vi "SSS_V4_0.vi"() -> ()   [LabVIEW 2017]
uses:
  <vilib>/DAQmx/write.llb/DAQmx Write (Analog 2D DBL NChan NSamp).vi
  <vilib>/DAQmx/read.llb/DAQmx Read (Analog 1D Wfm NChan NSamp).vi
  <vilib>/DAQmx/create/channels.llb/DAQmx Create Channel (AO-Voltage-Basic).vi
  <vilib>/DAQmx/create/channels.llb/DAQmx Create Channel (AI-Voltage-Basic).vi
  <vilib>/DAQmx/configure/timing.llb/DAQmx Timing (Sample Clock).vi
  <vilib>/DAQmx/miscellaneous.llb/DAQmx Fill In Error Info.vi
  <vilib>/Analysis/3filter.llb/FIR Filter (DBL).vi
  <vilib>/Analysis/NI_AALBase.lvlib
panel:
  out "크기 3":i32
  out "부호없는 바이트 배열":u8[](array[numeric])
  in  "Server Closed 2":string="The server VI closed the connection."
  out "연결 ID":refnum<k5>
  out "Signal Processing Result 2":waveform(dbl)(graph)
  out "Signal Processing Result":waveform(dbl)(graph)
  out "크기":i32
  in  "physical channels":tag="Dev3/ao0:1" caption="송신 채널 설정"
  in  "Samplig Rate(RX)":dbl=1500000.0
  in  "RX time(sec)":dbl=0.1
  out "RX.CH2":waveform(dbl)(graph)
  out "RX.CH1":waveform(dbl)(graph)
  in  "Start Frequency(Hz)":dbl=430000.0 format="%#_6p"
  in  "Pulse length(sec)":dbl=0.0004
  in  "sampling rate(TX)":dbl=3760000.0 caption="Sampling Rate(TX)" format="%#.2g"
  in  "STEP":i32=100
  in  "초기 위상":dbl format="%#_13g"
  in  "Bandwidth":dbl=40000.0 format="%#_6p"
  out "Hz/1STEP":dbl
  out "TX.CH1":waveform(dbl)(graph)
  out "TX.CH 2":waveform(dbl)(graph)
  in  "수신 디바이스 이름":tag="Dev3"
  in  "수신 채널 설정":tag="Dev3/ai0:1"
  in  "송신 디바이스 이름":tag="Dev3"
  out "불리언 2":bool
  in  "Signal_Processing 2":bool
  out "CMD_PWD_DATA":i32=4
  in  "Signal_Processing":bool
  out "CMD_PWD":i32=7
  out "CMD_TVG":i32=6
  out "CMD_TVG_DATA":i32=4
  out "CMD_GAIN":i32=5
  out "CMD_GAIN_DATA":i32=255
  out "CMD_RANGE":i32=4
  out "CMD_RANGE_DATA":i32=100
  out "CMD_STOP":i32=3
  out "CMD_STOP_DATA":i32
  out "CMD_START":i32=2
  out "CMD_START_DATA":i32=1
  in  "port":u16=2500
  in  "address":string="30.0.1.18"
  in  "TCP/IP":bool
  in  "Server Closed":string="The server VI closed the connection."
  # "송신 신호 변조 설정"
  # "DAQ Max 설정"
  # "TCP/IP 소켓 통신 설정"
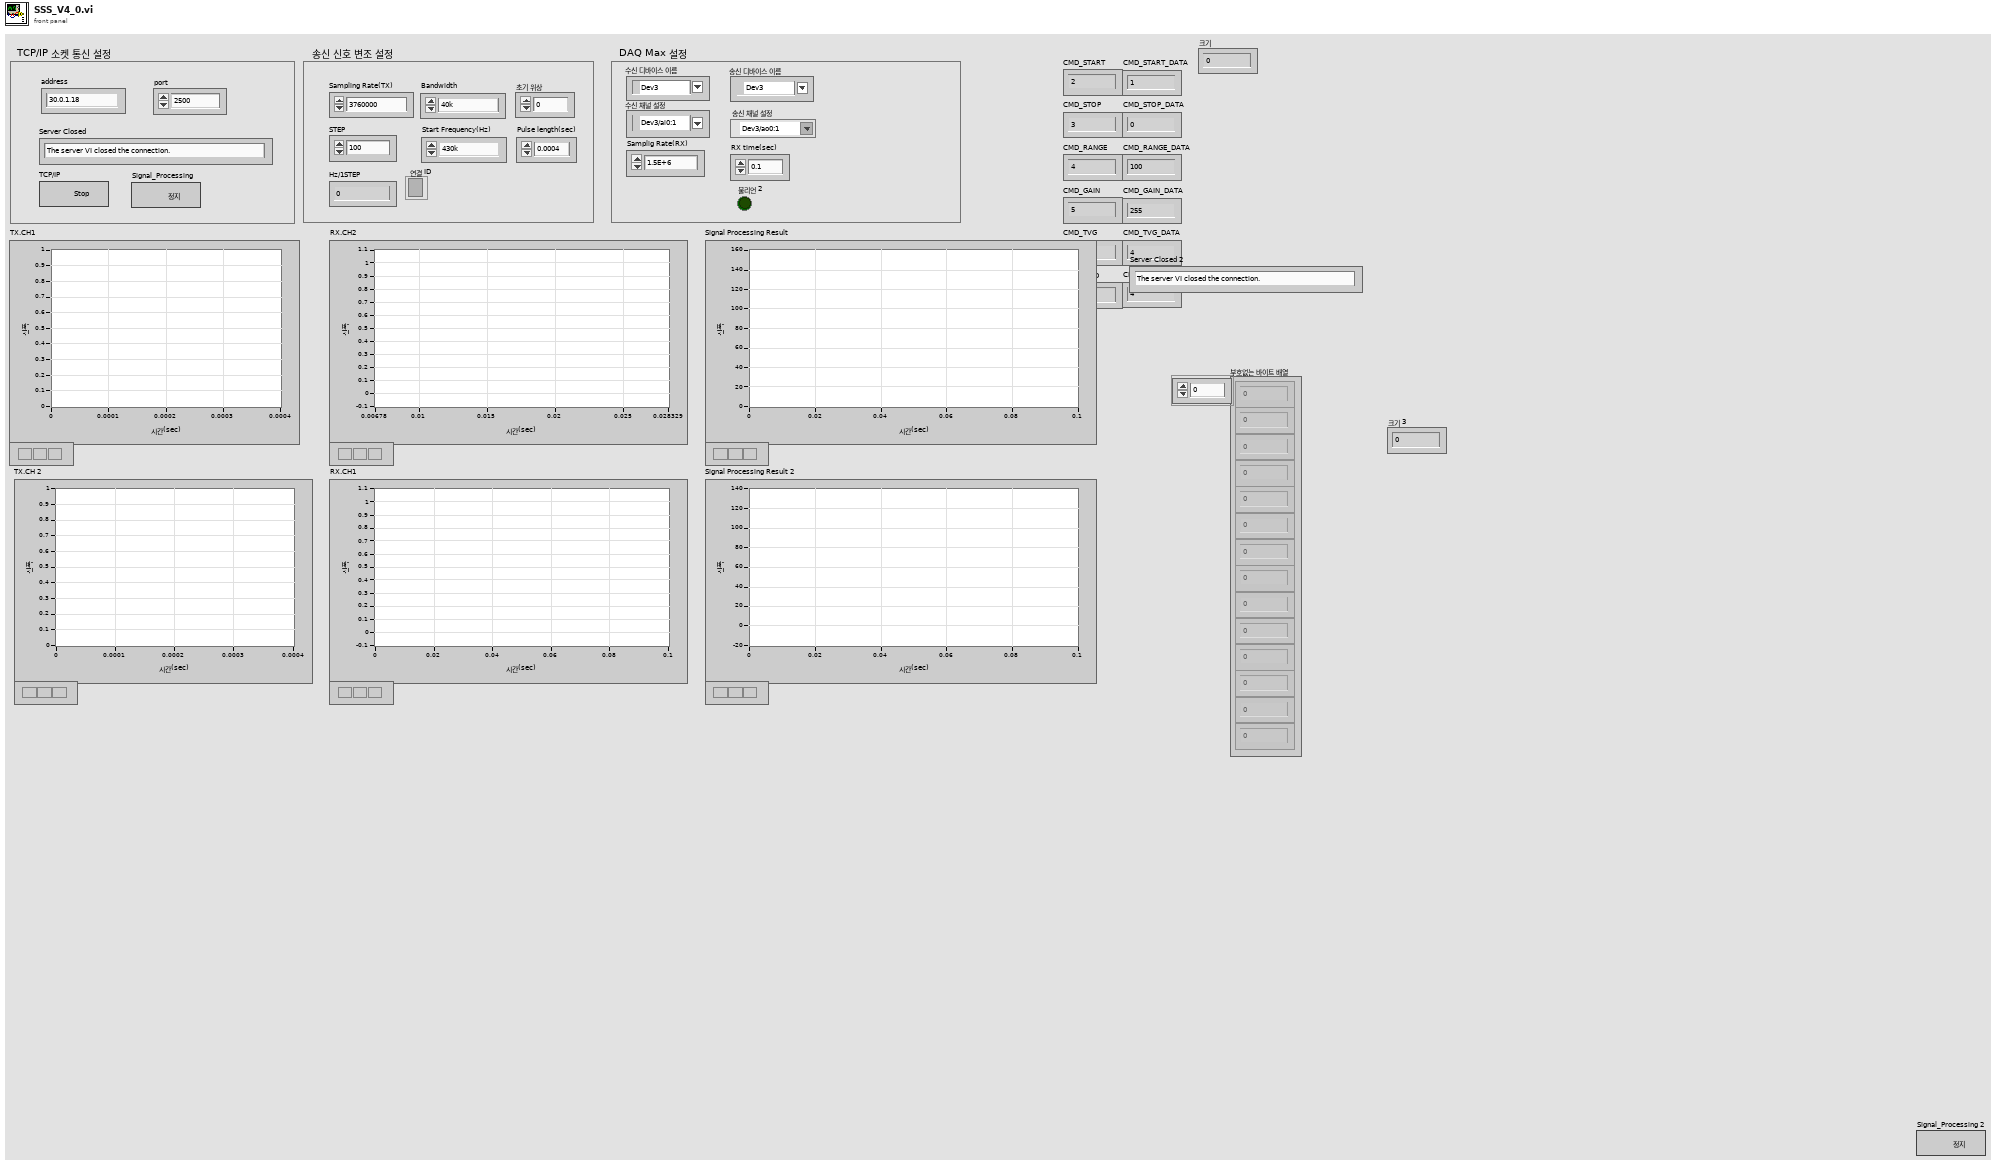
[diagram p1: front panel]
types:
  T1 = enum16{"Standard", "Buffered", "CRLF", "Immediate"}
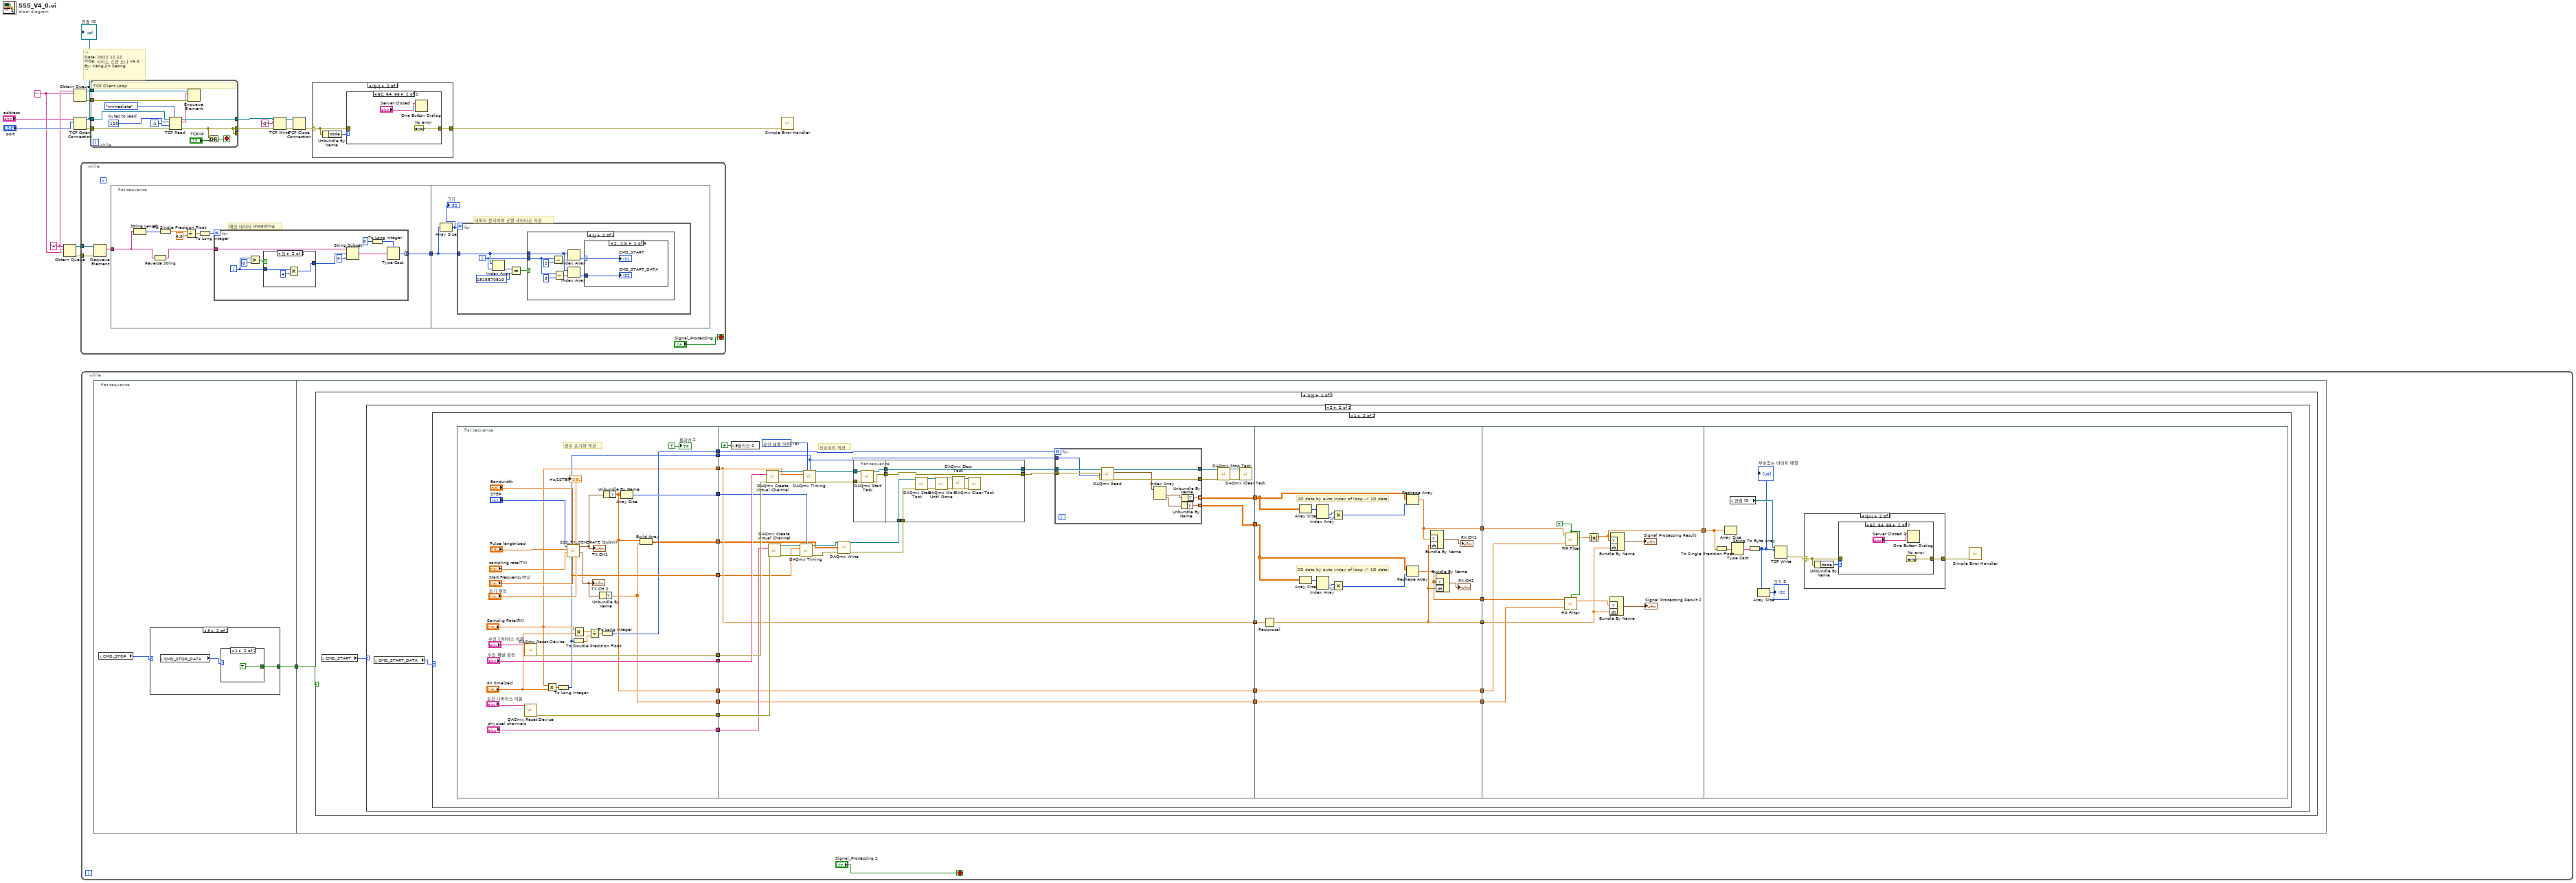
[diagram p0: block diagram]
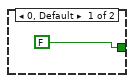
[diagram p2: hidden frame]
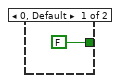
[diagram p3: hidden frame]
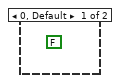
[diagram p4: hidden frame]
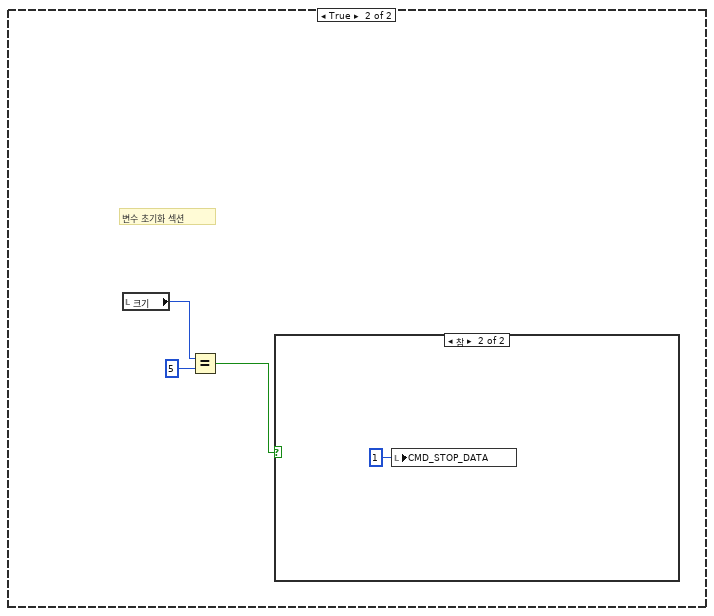
[diagram p8: hidden frame]
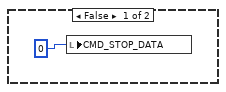
[diagram p9: hidden frame]
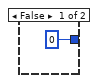
[diagram p10: hidden frame]
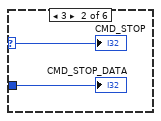
[diagram p12: hidden frame]
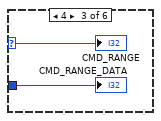
[diagram p13: hidden frame]
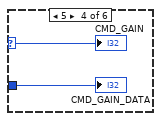
[diagram p14: hidden frame]
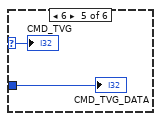
[diagram p15: hidden frame]
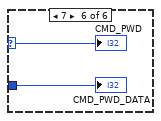
[diagram p16: hidden frame]
diagram:
  w1 = ""
  w4 = "A" ("이름(이름없음)")
  # "'''\nDate: 2022.12.12\nTitle: 사이드 스캔 소나 V4.0\nBy: Kang Jin Seong\n'''"
  n1 = Obtain Queue(name (unnamed)=w4, element data type=w1) -> (queue out=w3:refnum<queue>, error out=w2:errorcluster)  [unwired: 3 in, 1 out]
  n2 = Obtain Queue(name (unnamed)=w4, element data type=w1) -> (queue out=w6:refnum<queue>, error out=w5:errorcluster)  [unwired: 3 in, 1 out]
  n3 = TCP Open Connection(address="address", remote port or service name="port") -> (connection ID=w7:refnum<k5>, error out=w8:errorcluster)  [unwired: 3 in]
  "연결 ID" <- w7
  n4 = while {
    tunnel: w3 -> [w21]
    tunnel: w2 -> [w20]
    stop <- "Signal_Processing" stop-if-true
    n5 = Dequeue Element(queue=w21, error in (no error)=w20) -> (element=w19:string)  [unwired: 1 in, 3 out]
    n6 = flat-sequence {
      tunnel: w19 -> [w24]
      tunnel: [w25] -> w22
      tunnel: w22 -> [w45]
      frame #0 {
        # "패킷 데이터 Unpacking"
        n7 = String Length(string=w24) -> (length=w30:i32)
        n8 = Reverse String(1:w24) -> (0:w23:string)
        n9 = To Single Precision Float(number=w30) -> (single precision float=w29:sgl)
        n10 = Divide(x=w29, y=sgl 4.0) -> (x/y=w27:sgl)
        n11 = To Long Integer(number=w27) -> (32bit integer=w26:i32)
        n12 = for {
          N: w26 -> [_]
          tunnel: w23 -> [w40]
          tunnel: [w37] -> w25 mode=indexing
          i -> [w32]
          n13 = Greater?(x=w32, y=0) -> (0:w34:bool)
          n14 = case shown="참" w34 {
            tunnel: [0 w42] -> w33
            tunnel: w32 -> [_ w44]
            frame False {
            }
            frame True {
              n15 = Multiply(x=w44, y=4) -> (x*y=w42:i32)
            }
          }
          n16 = String Subset(string=w40, offset (0)=w33, length (rest)=4 ("길이(나머지)")) -> (substring=w31:string)
          n17 = To Long Integer(number=0 ("숫자")) -> (32bit integer=w39:i32)
          n18 = Type Cast(type=w39, x=w31) -> (*(type *) &x=w37:i32)
        }
      }
      frame #1 {
        # "데이터 분리하여 로컬 데이터로 저장"
        n19 = Array Size(array=w45) -> (size(s)=w46:i32)
        "크기" <- w46
        n20 = for {
          N: w46 -> [_]
          tunnel: w45 -> [w48]
          i -> [w47]
          n21 = Index Array(array=w48, index=w47) -> (element=w51:i32)
          n22 = Equal?(x=w51, y=1515870810) -> (x = y?=w49:bool)
          n23 = case shown="참" w49 {
            tunnel: w48 -> [_ w58]
            tunnel: w47 -> [_ w54]
            frame False {
            }
            frame True {
              n24 = Subtract(x=w54, y=2) -> (x-y=w52:i32)
              n25 = Subtract(x=w54, y=3) -> (x-y=w55:i32)
              n26 = Index Array(array=w58, index=w52) -> (element=w59:i32)
              n27 = Index Array(array=w58, index=w55) -> (element=w57:i32)
              n28 = case shown="2, 기본" w59 {
                selector: w59 -> [w61 w63 w65 w67 w69 w71]
                tunnel: w57 -> [w60 w62 w64 w66 w68 w70]
                frame 2, Default {
                  "CMD_START" <- w61
                  "CMD_START_DATA" <- w60
                }
                frame 3 {
                  "CMD_STOP" <- w63
                  "CMD_STOP_DATA" <- w62
                }
                frame 4 {
                  "CMD_RANGE" <- w65
                  "CMD_RANGE_DATA" <- w64
                }
                frame 5 {
                  "CMD_GAIN" <- w67
                  "CMD_GAIN_DATA" <- w66
                }
                frame 6 {
                  "CMD_TVG" <- w69
                  "CMD_TVG_DATA" <- w68
                }
                frame 7 {
                  "CMD_PWD" <- w71
                  "CMD_PWD_DATA" <- w70
                }
              }
            }
          }
        }
      }
    }
  }
  n29 = while {
    stop <- "Signal_Processing 2" stop-if-true
    n30 = flat-sequence {
      tunnel: [w74] -> w72
      tunnel: w72 -> [w81]
      frame #0 {
        n31 = local read "CMD_STOP"() -> (w75:i32)
        n32 = case shown="3" w75 {
          tunnel: [FALSE w77] -> w74
          frame 0, Default {
          }
          frame 3 {
            n33 = local read "CMD_STOP_DATA"() -> (w78:i32)
            n34 = case shown="1" w78 {
              tunnel: [FALSE TRUE] -> w77
              frame 0, Default {
              }
              frame 1 {
              }
            }
          }
        }
      }
      frame #1 {
        n35 = case shown="거짓" w81 {
          frame False {
            n36 = local read "CMD_START"() -> (w82:i32)
            n37 = case shown="2" w82 {
              frame 0, Default {
                (unwired) FALSE
              }
              frame 2 {
                n38 = local read "CMD_START_DATA"() -> (w83:i32)
                n39 = case shown="1" w83 {
                  frame 0, Default {
                  }
                  frame 1 {
                    n40 = flat-sequence {
                      tunnel: ["Start Frequency(Hz)"] -> w106
                      tunnel: ["수신 채널 설정"] -> w105
                      tunnel: [w121] -> w104
                      tunnel: ["Samplig Rate(RX)"] -> w103
                      tunnel: [w109] -> w102
                      tunnel: [w119] -> w101
                      tunnel: [w118] -> w100
                      tunnel: [w117] -> w99
                      tunnel: [w114] -> w95
                      tunnel: ["physical channels"] -> w94
                      tunnel: [w108] -> w92
                      tunnel: [w107] -> w90
                      tunnel: [w150] -> w98
                      tunnel: w106 -> [w140]
                      tunnel: w105 -> [w148]
                      tunnel: w104 -> [w147]
                      tunnel: w103 -> [w142]
                      tunnel: w102 -> [w141]
                      tunnel: w101 -> [w145]
                      tunnel: w100 -> [w144]
                      tunnel: w99 -> [w143]
                      tunnel: [w142] -> w97
                      tunnel: [w139] -> w96
                      tunnel: w95 -> [w137]
                      tunnel: w94 -> [w138]
                      tunnel: w92 -> [w136]
                      tunnel: [w136] -> w91
                      tunnel: w90 -> [w135]
                      tunnel: [w135] -> w89
                      tunnel: w98 -> [w205]
                      tunnel: w97 -> [w204]
                      tunnel: w96 -> [w199]
                      tunnel: [w197] -> w93
                      tunnel: w91 -> [w196]
                      tunnel: w89 -> [w195]
                      tunnel: [w196] -> w88
                      tunnel: [w195] -> w87
                      tunnel: [w194] -> w86
                      tunnel: [w193] -> w85
                      tunnel: w93 -> [w218]
                      tunnel: w88 -> [w212]
                      tunnel: w87 -> [w211]
                      tunnel: w86 -> [w217]
                      tunnel: w85 -> [w216]
                      tunnel: [w213] -> w84
                      tunnel: w84 -> [w225]
                      frame #0 {
                        # "변수 초기화 섹션"
                        n41 = call <vilib>:"DAQmx Reset Device.vi"("device in"="송신 디바이스 이름") -> ("error out"=w117:errorcluster)  [unwired: 1 in, 13 out]
                        n42 = call <vilib>:"DAQmx Reset Device.vi"("device in"="수신 디바이스 이름") -> ("error out"=w121:errorcluster)  [unwired: 1 in, 13 out]
                        n43 = Multiply(x="Samplig Rate(RX)", y="RX time(sec)") -> (x*y=w110:dbl)
                        n44 = To Long Integer(number=w110) -> (32bit integer=w109:i32)
                        n45 = call "SSS_TX_GENERATE (SubVI).vi"("초기 위상"="초기 위상", "Start Frequency(Hz)"="Start Frequency(Hz)", "Bandwidth"="Bandwidth", "sampling rate"="sampling rate(TX)", "Pulse length(sec)"="Pulse length(sec)", "STEP"="STEP") -> ("TX.CH1 2"=w115:waveform(dbl), "TX.CH1"=w120:waveform(dbl), "Hz/1STEP"=→"Hz/1STEP":dbl)  [unwired: 2 in, 1 out]
                        "TX.CH1" <- w120
                        "TX.CH 2" <- w115
                        n46 = To Double Precision Float(number=w109) -> (double precision float=w127:dbl)
                        n47 = Multiply(x="Samplig Rate(RX)", y="RX time(sec)") -> (x*y=w126:dbl)
                        n48 = Divide(x=w126, y=w127) -> (x/y=w128:dbl)
                        n49 = Unbundle By Name(w115) -> ("Y"=w107:dbl[])
                        n50 = To Long Integer(number=w128) -> (32bit integer=w118:i32)
                        n51 = Unbundle By Name(w120) -> ("Y"=w108:dbl[])
                        n52 = Array Size(array=w108) -> (size(s)=w119:i32)
                        n53 = Build Array(w108, w107) -> (w114:dbl[][])
                        "불리언 2" <- TRUE
                      }
                      frame #1 {
                        w146 = 10178 items=["유한 샘플"=10178, "연속 샘플"=10123, "하드웨어 타이밍에 의한 단일 포인트"=12522] ("sample mode")
                        # "신호처리 섹션"
                        n54 = local write "불리언 2"(FALSE) -> ()
                        n55 = call-poly <vilib>:"DAQmx Create Virtual Channel.vi"("physical channels"=w148, "error in"=w147) -> ("task out"=w165:refnum<k21>, "error out"=w166:errorcluster)  [unwired: 7 in, 5 out]
                        n56 = call-poly <vilib>:"DAQmx Create Virtual Channel.vi"("physical channels"=w138, "error in"=w143) -> ("task out"=w156:refnum<k21>, "error out"=w155:errorcluster)  [unwired: 7 in, 5 out]
                        n57 = call-poly <vilib>:"DAQmx Timing.vi"("task/channels in"=w156, "samples per channel"=w145, "rate"=w140, "error in"=w155) -> ("task out"=w153:refnum<k21>, "error out"=w154:errorcluster)  [unwired: 3 in, 7 out]
                        n58 = call-poly <vilib>:"DAQmx Timing.vi"("task/channels in"=w165, "sample mode"=w146, "samples per channel"=w141, "rate"=w142, "error in"=w166) -> ("task out"=w164:refnum<k21>, "error out"=w163:errorcluster)  [unwired: 2 in, 7 out]
                        n59 = call-poly <vilib>:"DAQmx Write.vi"("task/channels in"=w153, "data"=w137, "error in"=w154) -> ("task out"=w152:refnum<k21>, "error out"=w151:errorcluster)  [unwired: 10 in, 1 out]
                        n60 = flat-sequence {
                          tunnel: [w182] -> w168
                          tunnel: [w181] -> w167
                          tunnel: w164 -> [w180]
                          tunnel: w163 -> [w179]
                          tunnel: w168 -> [w192]
                          tunnel: [w192] -> w161
                          tunnel: [w191] -> w162
                          tunnel: w167 -> [w191]
                          tunnel: w152 -> [w190]
                          tunnel: w151 -> [w189]
                          frame #0 {
                            n61 = call <vilib>:"DAQmx Start Task.vi"("task/channels in"=w180, "error in"=w179) -> ("task out"=w181:refnum<k21>, "error out"=w182:errorcluster)  [unwired: 12 in]
                          }
                          frame #1 {
                            n62 = call <vilib>:"DAQmx Start Task.vi"("task/channels in"=w190, "error in"=w189) -> ("task out"=w183:refnum<k21>, "error out"=w188:errorcluster)  [unwired: 12 in]
                            n63 = call <vilib>:"DAQmx Wait Until Done.vi"("task/channels in"=w183, "error in"=w188) -> ("task out"=w184:refnum<k21>, "error out"=w187:errorcluster)  [unwired: 12 in]
                            n64 = call <vilib>:"DAQmx Stop Task.vi"("task/channels in"=w184, "error in"=w187) -> ("task out"=w185:refnum<k21>, "error out"=w186:errorcluster)  [unwired: 12 in]
                            n65 = call <vilib>:"DAQmx Clear Task.vi"("task in"=w185, "error in"=w186) -> ()  [unwired: 13 in, 1 out]
                          }
                        }
                        n66 = for {
                          N: w144 -> [_]
                          tunnel: w162 -> [w178]
                          tunnel: w161 -> [w177]
                          tunnel: [w176] -> w160
                          tunnel: [w175] -> w157
                          tunnel: [w174] -> w150 mode=indexing
                          tunnel: w141 -> [w173]
                          tunnel: [w169] -> w139 mode=indexing
                          n67 = call-poly <vilib>:"DAQmx Read.vi"("task/channels in"=w178, "number of samples per channel"=w173, "error in"=w177) -> ("task out"=w175:refnum<k21>, "data"=w172:waveform(dbl)[], "error out"=w176:errorcluster)  [unwired: 10 out]
                          n68 = Index Array(array=w172) -> (element #1=w171:waveform(dbl), element #2=w170:waveform(dbl))  [unwired: 2 in]
                          n69 = Unbundle By Name(w170) -> ("Y"=w169:dbl[])
                          n70 = Unbundle By Name(w171) -> ("Y"=w174:dbl[])
                        }
                        n71 = call <vilib>:"DAQmx Stop Task.vi"("task/channels in"=w157, "error in"=w160) -> ("task out"=w158:refnum<k21>, "error out"=w159:errorcluster)  [unwired: 12 out]
                        n72 = call <vilib>:"DAQmx Clear Task.vi"("task in"=w158, "error in"=w159) -> ()  [unwired: 14 out]
                      }
                      frame #2 {
                        # "2D data by auto index of loop -> 1D data"
                        # "2D data by auto index of loop -> 1D data"
                        n73 = Reciprocal(x=w204) -> (1/x=w197:dbl)
                        n74 = Array Size(array=w205) -> (size(s)=w208:i32[])
                        n75 = Array Size(array=w199) -> (size(s)=w201:i32[])
                        n76 = Index Array(array=w208) -> (element #1=w209:i32, element #2=w206:i32)  [unwired: 2 in]
                        n77 = Index Array(array=w201) -> (element #1=w202:i32, element #2=w200:i32)  [unwired: 2 in]
                        n78 = Multiply(x=w209, y=w206) -> (x*y=w210:i32)
                        n79 = Multiply(x=w202, y=w200) -> (x*y=w203:i32)
                        n80 = Reshape Array(w205, w210) -> (w194:dbl[])
                        n81 = Reshape Array(w199, w203) -> (w193:dbl[])
                        n82 = Bundle By Name("Y"=w194, "dt"=w197) -> (→"RX.CH1":waveform(dbl))  [unwired: 1 in]
                        n83 = Bundle By Name("Y"=w193, "dt"=w197) -> (→"RX.CH2":waveform(dbl))  [unwired: 1 in]
                      }
                      frame #3 {
                        w221 = TRUE ("init/cont (init:F)")
                        n84 = call-poly <vilib>:"FIR Filter.vi"("init/cont (init:F)"=w221, "FIR Coefficients"=w211, "X"=w216) -> ("Filtered X"=w220:dbl[])  [unwired: 1 in, 1 out]
                        n85 = call-poly <vilib>:"FIR Filter.vi"("init/cont (init:F)"=w221, "FIR Coefficients"=w212, "X"=w217) -> ("Filtered X"=w219:dbl[])  [unwired: 1 in, 1 out]
                        n86 = Absolute Value(x=w219) -> (abs(x)=w213:dbl[])
                        n87 = Bundle By Name("Y"=w220, "dt"=w218) -> (→"Signal Processing Result 2":waveform(dbl))  [unwired: 1 in]
                        n88 = Bundle By Name("Y"=w213, "dt"=w218) -> (→"Signal Processing Result":waveform(dbl))  [unwired: 1 in]
                      }
                      frame #4 {
                        n89 = To Single Precision Float(number=w225) -> (single precision float=w229:sgl[])
                        n90 = Array Size(array=w225) -> ()  [unwired: 1 out]
                        n91 = local read "연결 ID"() -> (w228:refnum<k5>)
                        n92 = Type Cast(x=w229) -> (*(type *) &x=w222:string)  [unwired: 1 in]
                        n93 = String To Byte Array(string=w222) -> (unsigned byte array=w224:u8[])
                        "부호없는 바이트 배열" <- w224
                        n94 = Array Size(array=w224) -> (size(s)=→"크기 3":i32)
                        n95 = TCP Write(connection ID=w228, data in=w224) -> (error out=w226:errorcluster)  [unwired: 2 in, 2 out]
                        n96 = case shown="에러" w226 {
                          selector: w226 -> [w230 w232]
                          tunnel: [w230 w231] -> w227
                          frame No Error {
                          }
                          frame Error {
                            n97 = Unbundle By Name(w232) -> ("code"=w233:i32)
                            n98 = case shown="62, 64, 66" w233 {
                              tunnel: w232 -> [w234 _]
                              tunnel: [w234 w236] -> w231
                              frame Default {
                              }
                              frame 62, 64, 66 {
                                w236 = errorcluster {"status"=FALSE, "code"=0, "source"=""}  # No error
                                n99 = One Button Dialog(message="Server Closed 2") -> ()  [unwired: 1 in, 1 out]
                              }
                            }
                          }
                        }
                        n100 = call <vilib>:"Simple Error Handler.vi"("error in (no error)"=w227) -> ()  [unwired: 4 in, 5 out]
                      }
                    }
                  }
                }
              }
            }
          }
          frame True {
            # "변수 초기화 섹션"
            n101 = local read "크기"() -> (w238:i32)
            n102 = Equal?(x=w238, y=5) -> (x = y?=w237:bool)
            n103 = case shown="참" w237 {
              frame False {
                n104 = local write "CMD_STOP_DATA"(0) -> ()
              }
              frame True {
                n105 = local write "CMD_STOP_DATA"(1 ("CMD_STOP_DATA")) -> ()
              }
            }
          }
        }
      }
    }
  }
  n106 = while {
    tunnel: [w251] -> w16
    tunnel: [w244] -> w14
    tunnel: w8 -> [w249]
    tunnel: w7 -> [w248]
    tunnel: w6 -> [w247]
    tunnel: w5 -> [w246]
    tunnel: [w244] -> _
    stop <- w252 stop-if-true
    w253 = 120  # bytes to read
    # "TCP Client Loop"
    n107 = TCP Read(connection ID=w248, bytes to read=w253, error in (no error)=w249, 7:T1."Immediate" ("모드(standard)"), 9:-1 ("타임아웃 ms (25000)")) -> (connection ID out=w251:refnum<k5>, data out=w242:string, error out=w244:errorcluster)
    n108 = Enqueue Element(queue=w247, element=w242, error in (no error)=w246) -> ()  [unwired: 1 in, 3 out]
    n109 = Or(x=w244, y="TCP/IP") -> (x .or. y?=w252:bool)
  }
  n110 = TCP Write(connection ID=w16, data in="Q", error in (no error)=w14) -> (connection ID out=w17:refnum<k5>, error out=w15:errorcluster)  [unwired: 2 out]
  n111 = TCP Close Connection(connection ID=w17, error in (no error)=w15) -> (error out=w12:errorcluster)  [unwired: 1 in, 1 out]
  n112 = case shown="에러" w12 {
    selector: w12 -> [w254 w256]
    tunnel: [w254 w255] -> w11
    frame No Error {
    }
    frame Error {
      n113 = Unbundle By Name(w256) -> ("code"=w257:i32)
      n114 = case shown="62, 64, 66" w257 {
        tunnel: w256 -> [w258 _]
        tunnel: [w258 w260] -> w255
        frame Default {
        }
        frame 62, 64, 66 {
          w260 = errorcluster {"status"=FALSE, "code"=0, "source"=""}  # No error
          n115 = One Button Dialog(message="Server Closed") -> ()  [unwired: 1 in, 1 out]
        }
      }
    }
  }
  n116 = call <vilib>:"Simple Error Handler.vi"("error in (no error)"=w11) -> ()  [unwired: 4 in, 5 out]
